vi "get_description.vi"(8 "error in (no error)":errorcluster, 11 "Mocha in":refnum<class "Mocha.lvclass">) -> (0 "error out":errorcluster, 2 "Description":string, 3 "Mocha out":refnum<class "Mocha.lvclass">)   [LabVIEW 2021, in "Mocha.lvclass"]
uses:
  Mocha.lvclass
  Beverage/Beverage.lvclass
  Mocha.lvclass/Mocha.ctl
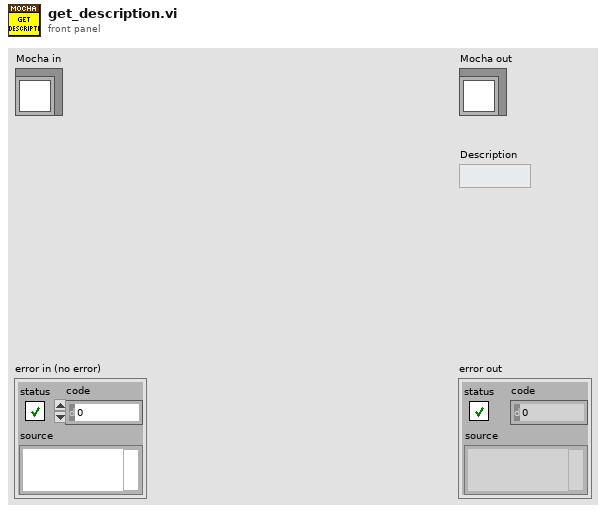
[diagram p1: front panel]
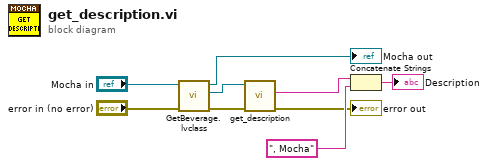
[diagram p0: block diagram]
diagram:
  n1 = call-dynamic "GetBeverage.lvclass.vi"("error in (no error)"="error in (no error)", "object in"="Mocha in") -> ("error out"=w2:errorcluster, "Beverage.lvclass"=w5:refnum<class "Beverage.lvclass">, "object out"=→"Mocha out":refnum<class "Mocha.lvclass">)  [unwired: 7 in]
  n2 = call-dynamic "get_description.vi"("error in (no error)"=w2, "Beverage in"=w5) -> ("error out"=→"error out":errorcluster, "Description"=w1:string)  [unwired: 7 in, 1 out]
  n3 = Concatenate Strings(w1, ", Mocha" ("string")) -> (→"Description":string)
